vi "Play Path.vi"(7 "Description":string, 8 "Command Info In":T3, 10 "Synchronization":enum16{"Start", "Wait"}(ring), 11 "Auto Data":T2) -> (0 "Command Info Out":T3)   [LabVIEW 2023]
doc: "This VI notifies the subsystem to the new setpoint."
uses:
  <vilib>/Rock Robotics/WPI/Framework/Command Status Info.ctl
  <vilib>/Rock Robotics/WPI/Framework/Completion Status.ctl
  <vilib>/Rock Robotics/WPI/Framework/Completion Notifier.ctl
  swerve/Type Definitions/Data/Robot Velocities.ctl
  Implementation/Drive Setpoints.ctl
  Implementation/Drive Operations.ctl
  Framework/Robot Global Data.vi
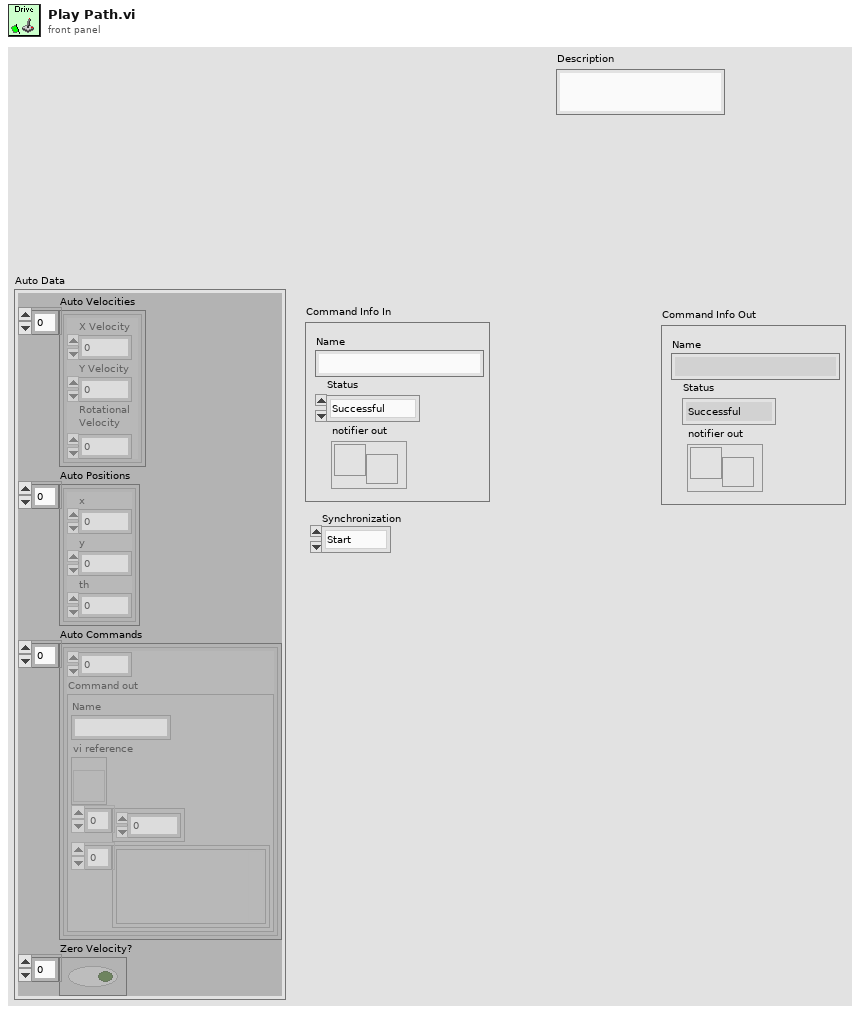
[diagram p1: front panel]
types:
  T1 = typedef "Robot Velocities.ctl" = cluster{"X Velocity":dbl, "Y Velocity":dbl, "Rotational \nVelocity":dbl}
  T2 = cluster{"Auto Velocities":T1[], "Auto Positions":cluster{"x":dbl, "y":dbl, "th":dbl}[], "Auto Commands":cluster{dbl, "Command out":cluster{"Name":string, "vi reference":refnum<vi>, i32[], variant[]}}[], "Zero Velocity?":bool[]}
  T3 = typedef "Command Status Info.ctl" = cluster{"Name":string, "Status":T4, "notifier out":T5}
  T4 = typedef "Completion Status.ctl" = enum16{"Successful", "Aborted", "Incomplete"}
  T5 = typedef "Completion Notifier.ctl" = refnum<notifier>
  T6 = typedef "Drive Setpoints.ctl" = cluster{"Operation":T7, "Robot Velocities":T1, "Auto Data":cluster{"Auto Velocities":T1[], "Auto Positions":cluster{"x":dbl, "y":dbl, "th":dbl}[], "Auto Commands":cluster{dbl, "Command out":cluster{"Name":string, "vi reference":refnum<vi>, i32[], variant[]}}[], "Zero Velocity?":bool[]}, "Left side":bool, "Angle Align":bool, "Tag ID":i32}
  T7 = typedef "Drive Operations.ctl" = enum16{"Reserve", "Read Current", "Immediate", "Calibrate", "Reef Align", "Auto"}
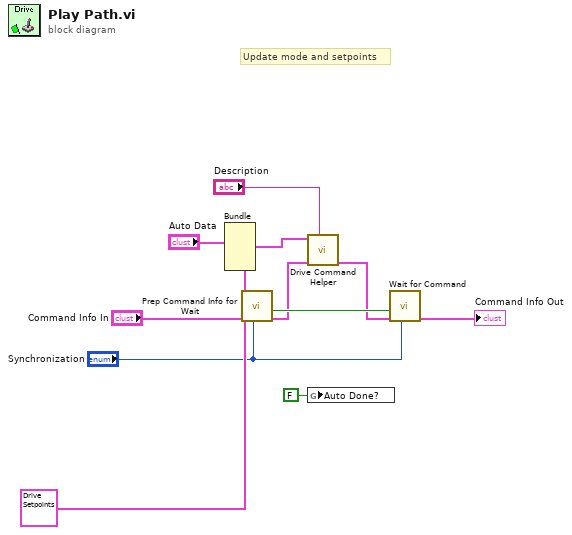
[diagram p0: block diagram]
diagram:
  # "Update mode and setpoints"
  n1 = Bundle(cluster=T6 {"Operation"=enum."Auto", "Robot Velocities"={"X Velocity"=0.0, "Y Velocity"=0.0, "Rotational \nVelocity"=0.0}, "Auto Data"={"Auto Velocities"=[], "Auto Positions"=[], "Auto Commands"=[], "Zero Velocity?"=[]}, "Left side"=FALSE, "Angle Align"=FALSE, "Tag ID"=0} ("SubSystem Data"), "Auto Data"="Auto Data") -> (w10:T6)  [unwired: 5 in]
  n2 = call <vilib>:"Prep Command Info for Wait.vi"("Synchronication"="Synchronization", "Command Info"="Command Info In") -> ("Command Info"=w5:T3, "Allocated"=w8:bool)  [unwired: 8 in]
  n3 = call "Drive Command Helper.vi"("Description"="Description", "Command Info In"=w5, "SubSystem Data"=w10) -> ("Command Info Out"=w4:T3)  [unwired: 6 in, 2 out]
  n4 = global write "Robot Global Data.vi" "Auto Done?"(FALSE ("Auto Done?")) -> ()
  n5 = call <vilib>:"Wait for Command.vi"("Synchronication"="Synchronization", "Command Info in"=w4, "Allocated"=w8) -> ("Command Info out"=→"Command Info Out":T3)  [unwired: 8 in]
